vi "Create All Message Queues.vi"(8 "error in (no error)":errorcluster, 11 "Share_Data":T1 {"ConfigurationDatabase"."InactivityTime" format="%.0f seconds"; "ConfigurationDatabase"."TravelTime" format="%.0f seconds"; "ConfigurationDatabase"."DoorClose" format="%.0f seconds"; "ConfigurationDatabase"."DoorOpen" format="%.0f seconds"}) -> (0 "error out":errorcluster, 3 "Message Queues out":T4)   [LabVIEW 2020, in "Message Queue.lvlib"]
doc: "This VI creates and initializes all the message queues for your application. If your application requires more than one message queue, right-click the \"Message Queues\" constant above and select Open Type Def. Add the new Message Queue(s) to the type definition, then initialize them in this VI."
uses:
  Message Queue.lvlib
  All Message Queues.ctl
  Message Cluster.ctl
  controls/Share_Data.ctl
  controls/Configuration_Database.ctl
  controls/Event_User.ctl
  Enqueue Message (Single).vi
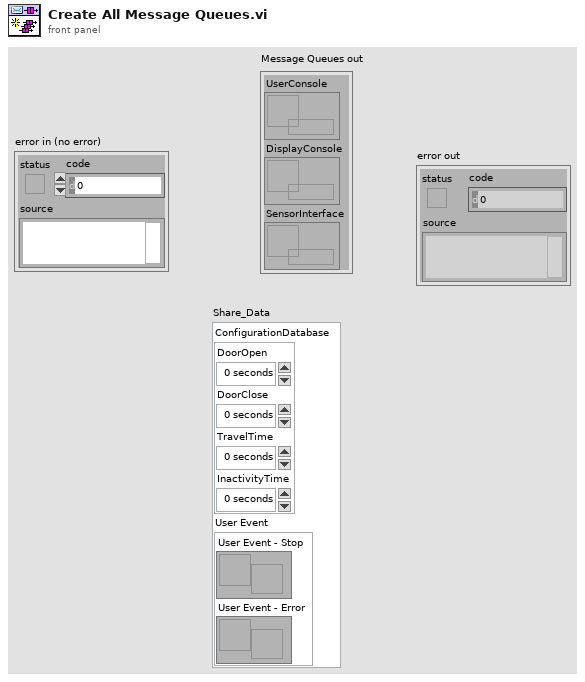
[diagram p1: front panel]
types:
  T1 = typedef "Share_Data.ctl" = cluster{"ConfigurationDatabase":T2, "User Event":T3}
  T2 = typedef "Configuration_Database.ctl" = cluster{"DoorOpen":u8, "DoorClose":u8, "TravelTime":u8, "InactivityTime":u8}
  T3 = typedef "Event_User.ctl" = cluster{"User Event - Stop":refnum<user-event>, "User Event - Error":refnum<user-event>}
  T4 = typedef "Message Queue.lvlib/All Message Queues.ctl" = cluster{"UserConsole":refnum<queue>, "DisplayConsole":refnum<queue>, "SensorInterface":refnum<queue>}
  T5 = cluster{"[0]":refnum<queue>, "[1]":refnum<queue>, "[2]":refnum<queue>}
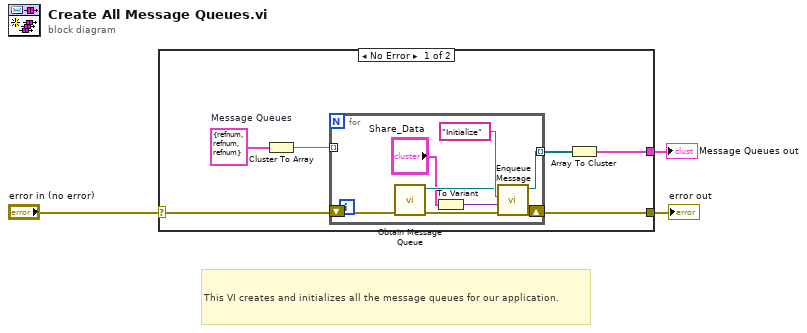
[diagram p0: block diagram]
diagram:
  # "This VI creates and initializes all the message queues for our application."
  n1 = case shown="No Error" "error in (no error)" {
    selector: "error in (no error)" -> [w8 w18]
    tunnel: [w9 w18] -> w3
    tunnel: [w4 _] -> w2
    frame No Error {
      w7 = T4 {"UserConsole"=refnum, "DisplayConsole"=refnum, "SensorInterface"=refnum}  # Message Queues
      n2 = Cluster To Array(cluster=w7) -> (array=w6:refnum<queue>[])
      n3 = for {
        shift-right: [w17] -> w9
        shift-left: w8 -> [w16]
        tunnel: w6 -> [_] mode=indexing
        tunnel: [w12] -> w5 mode=indexing
        n4 = call "Obtain Message Queue.vi"("error in (no error)"=w16) -> ("error out"=w15:errorcluster, "Message Queue"=w13:refnum<queue>)  [unwired: 9 in]
        n5 = To Variant(anything="Share_Data") -> (Variant=w10:variant)
        n6 = call-poly "Enqueue Message.vi"("error in (no error)"=w15, "Message Data"=w10, "Message"="Initialize", "Message Queue"=w13) -> ("error out"=w17:errorcluster, "dup Message Queue"=w12:refnum<queue>)  [unwired: 6 in]
      }
      n7 = Array To Cluster(array=w5) -> (cluster=w4:T5)
    }
    frame Error {
    }
  }
  "Message Queues out" <- w2
  "error out" <- w3
